vi "Initialize.vi"(8 "error in (no error)":errorcluster, 11 "HOTCOIL Settings":T1) -> (0 "error out":errorcluster, 2 "Connection Error":bool, 3 "HOTCOIL Settings":T1)   [LabVIEW 2021, in "HotCoil.lvlib"]
uses:
  HotCoil.lvlib
  HotCoil Settings.ctl
  <vilib>/Instr/_visa.llb/VISA Configure Serial Port (Instr).vi
panel:
  out "Array":string[](array[string])
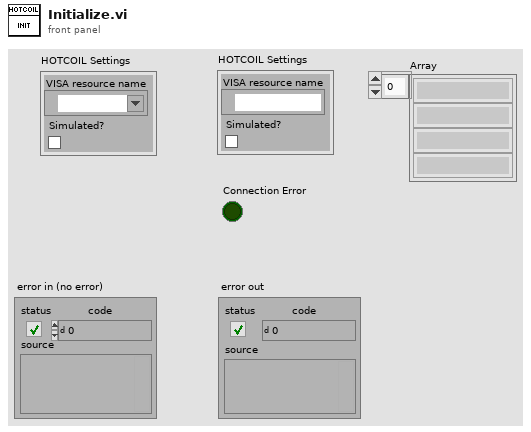
[diagram p1: front panel]
types:
  T1 = typedef "HotCoil.lvlib/HotCoil Settings.ctl" = cluster{"VISA resource name":refnum<visa-resource-name>, "Simulated?":bool}
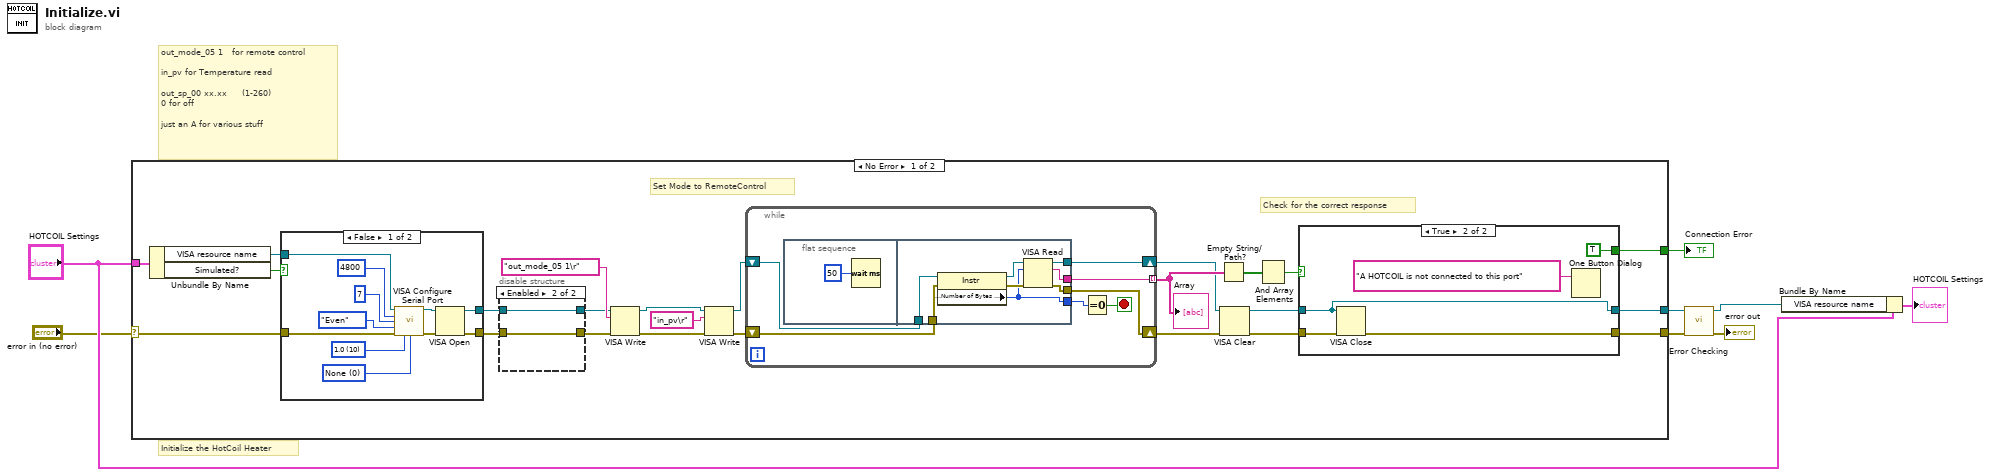
[diagram p0: block diagram]
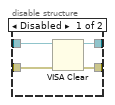
[diagram p2: hidden frame]
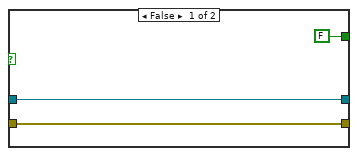
[diagram p3: hidden frame]
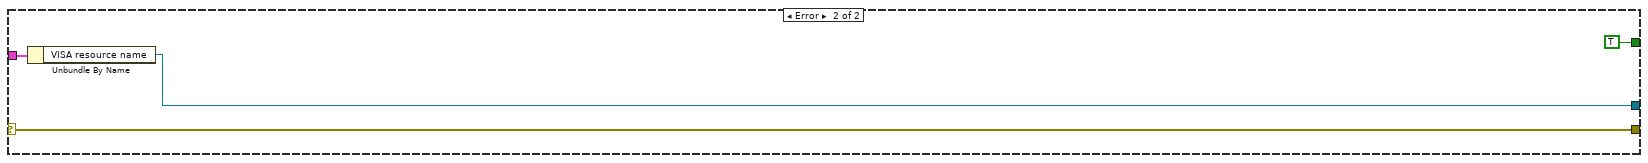
[diagram p5: hidden frame]
diagram:
  # "out_mode_05 1   for remote control\n\nin_pv for Temperature read\n\nout_sp_00 xx.xx     (1-260)\n0 for off\n\njust an A for various stuff"
  # "Initialize the HotCoil Heater"
  n1 = case shown="No Error" "error in (no error)" {
    selector: "error in (no error)" -> [w32 w79]
    tunnel: "HOTCOIL Settings" -> [w30 w78]
    tunnel: [w27 w79] -> w6
    tunnel: [w28 w77] -> w8
    tunnel: [w24 TRUE] -> w2
    frame No Error {
      # "Check for the correct response"
      # "Set Mode to RemoteControl"
      n2 = Unbundle By Name(w30) -> ("VISA resource name"=w29:refnum<visa-resource-name>, "Simulated?"=w31:bool)
      n3 = case shown="False" w31 {
        tunnel: w32 -> [w67 w75]
        tunnel: [w63 w75] -> w18
        tunnel: [w64 w74] -> w19
        tunnel: w29 -> [w65 w74]
        frame False {
          w69 = u16 0 items=["None", "XON/XOFF", "RTS/CTS", "XON/XOFF & RTS/CTS", "DTR/DSR", "XON/XOFF & DTR/DSR"] ("flow control (0:none)")
          w70 = u16 10 items=["1.0"=10, "1.5"=15, "2.0"=20] ("stop bits (10: 1 bit)")
          n4 = call-poly "VISA Configure Serial Port"("VISA resource name"=w65, "baud rate (9600)"=u32 4800, "data bits (8)"=u16 7, "parity (0:none)"=enum16{"None", "Odd", "Even", "Mark", "Space"}."Even", "error in (no error)"=w67, "stop bits (10: 1 bit)"=w70, "flow control (0:none)"=w69) -> ("VISA resource name out"=w66:refnum<visa-resource-name>, "error out"=w68:errorcluster)  [unwired: 7 in]
          n5 = VISA Open(error in (no error)=w68, VISA resource name=w66) -> (VISA resource name=w64:refnum<visa-resource-name>, error out=w63:errorcluster)  [unwired: 3 in]
        }
        frame True {
        }
      }
      n6 = disable-structure shown="Enabled" {
        disable-tunnel: w19 -> [w36 w38]
        disable-tunnel: w18 -> [w35 w37]
        disable-tunnel: [w34 w38] -> w17
        disable-tunnel: [w33 w37] -> w16
        frame Disabled {
          n7 = VISA Clear(VISA resource name=w36, error in (no error)=w35) -> (VISA resource name out=w34:refnum<visa-resource-name>, error out=w33:errorcluster)
        }
        frame Enabled {
        }
      }
      n8 = VISA Write(VISA resource name=w17, write buffer="out_mode_05 1\r", error in (no error)=w16) -> (VISA resource name out=w13:refnum<visa-resource-name>, error out=w12:errorcluster)  [unwired: 1 out]
      n9 = VISA Write(VISA resource name=w13, write buffer="in_pv\r", error in (no error)=w12) -> (VISA resource name out=w10:refnum<visa-resource-name>, error out=w9:errorcluster)  [unwired: 1 out]
      n10 = while {
        shift-right: [w45] -> w15
        shift-left: w10 -> [w40]
        shift-right: [w44] -> w14
        shift-left: w9 -> [w39]
        tunnel: [w41] -> w22 mode=indexing
        stop <- w42 stop-if-true
        n11 = flat-sequence {
          tunnel: [w54] -> w44
          tunnel: [w53] -> w41
          tunnel: [w52] -> w45
          tunnel: [w47] -> w43
          tunnel: w40 -> [w51]
          tunnel: w39 -> [w50]
          frame #0 {
            n12 = Wait (ms)(milliseconds to wait=u32 50) -> ()  [unwired: 1 out]
          }
          frame #1 {
            n13 = property class="Instr"(reference=w51, error in=w50) -> (reference out=w49:refnum<visa-resource-name>, error out=w48:errorcluster, "Serial Settings:Number of Bytes at Serial Port"=w47:u32)
            n14 = VISA Read(VISA resource name=w49, byte count=w47, error in (no error)=w48) -> (VISA resource name out=w52:refnum<visa-resource-name>, read buffer=w53:string, error out=w54:errorcluster)  [unwired: 1 out]
          }
        }
        n15 = Equal To 0?(x=w43) -> (x = 0?=w42:bool)
      }
      "Array" <- w22
      n16 = Empty String/Path?(string/path=w22) -> (empty?=w20:bool[])
      n17 = VISA Clear(VISA resource name=w15, error in (no error)=w14) -> (VISA resource name out=w26:refnum<visa-resource-name>, error out=w25:errorcluster)
      n18 = And Array Elements(Boolean array=w20) -> (logical AND=w21:bool)
      n19 = case shown="True" w21 {
        tunnel: w26 -> [w57 w60]
        tunnel: w25 -> [w56 w61]
        tunnel: [w57 w60] -> w28
        tunnel: [w56 w59] -> w27
        tunnel: [FALSE TRUE] -> w24
        frame False {
        }
        frame True {
          n20 = VISA Close(VISA resource name=w60, error in (no error)=w61) -> (error out=w59:errorcluster)
          n21 = One Button Dialog(message="A HOTCOIL is not connected to this port") -> ()  [unwired: 1 in, 1 out]
        }
      }
    }
    frame Error {
      n22 = Unbundle By Name(w78) -> ("VISA resource name"=w77:refnum<visa-resource-name>)
    }
  }
  "Connection Error" <- w2
  n23 = call "Error Checking.vi"("error in (no error)"=w6, "VISA resource name"=w8) -> ("error out"=→"error out":errorcluster, "VISA resource name"=w7:refnum<visa-resource-name>)  [unwired: 7 in, 1 out]
  n24 = Bundle By Name(cluster="HOTCOIL Settings", "VISA resource name"=w7) -> (→"HOTCOIL Settings":T1)
